vi "S2C_Shared_Proc_GetClusterValues.vi"(4 "LabelText":string, 6 "ClassName":string, 8 "Error In":errorcluster, 9 "CtrlRef":refnum<vi>) -> (0 "Error Out":errorcluster, 2 "Valid?":bool, 3 "Settings":string[](array[string]))   [LabVIEW 2024]
uses:
  <vilib>/Utility/Data Type/NI_Data Type.lvlib
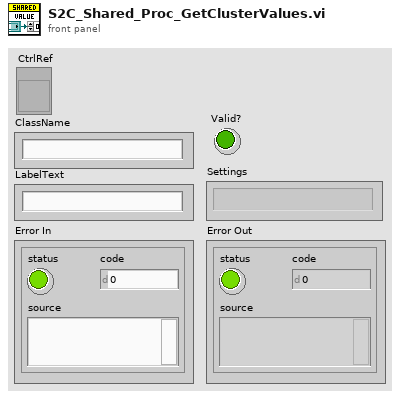
[diagram p1: front panel]
types:
  T1 = typedef "NI_Data Type.lvlib/Data Type.ctl" = enum8{"Invalid Type", "Void", "I8", "I16", "I32", "I64", "U8", "U16", "U32", "U64", "Single Float", "Double Float", "Extended Float", "Single Complex", "Double Complex", "Extended Complex", "Enum U8", "Enum U16", "Enum U32", "Enum U64", "Single Float With Unit", "Double Float With Unit", "Extended Float With Unit", "Single Complex with Unit", "Double Complex with Unit", "Extended Complex with Unit", "Boolean", "String", "Path", "Picture", "Tag", "Array", "Cluster", "Variant", "LV Variant", "Waveform", "Timestamp", "Digital Waveform", "Digital Data", "ExpressData", "Refnum", "External Data", "VI", "Poly VI", "LabVIEW Class Instance", "Fixed Point", "Set Collection", "Map Collection"}
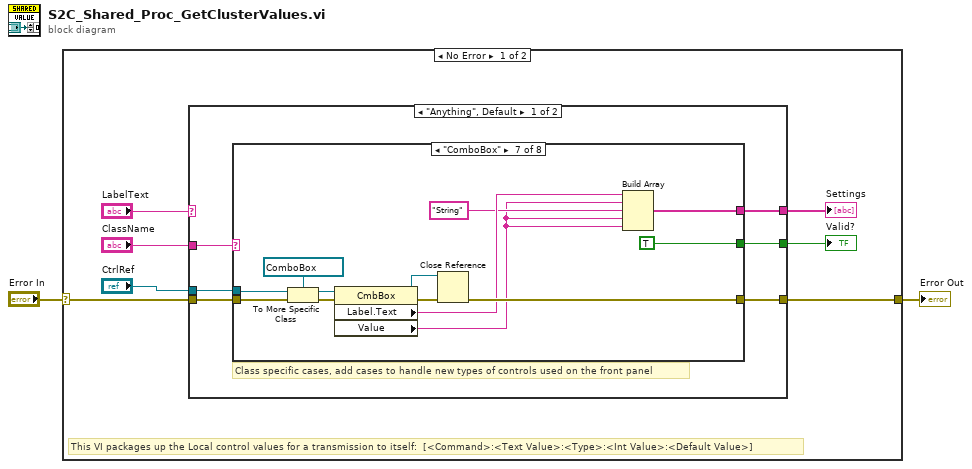
[diagram p0: block diagram]
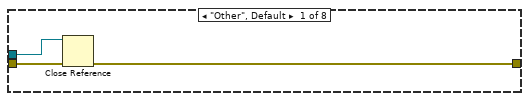
[diagram p2: hidden frame]
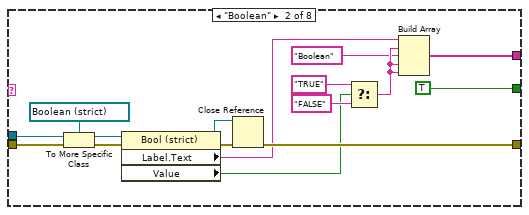
[diagram p3: hidden frame]
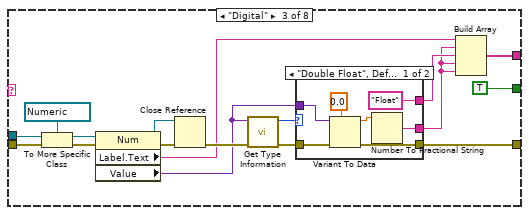
[diagram p4: hidden frame]
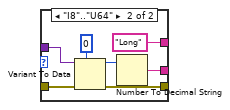
[diagram p5: hidden frame]
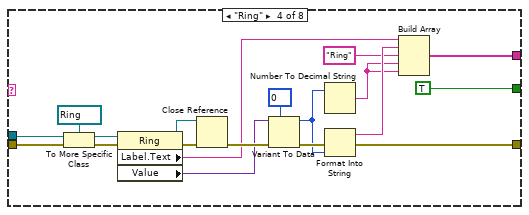
[diagram p6: hidden frame]
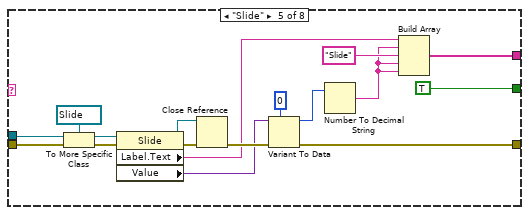
[diagram p7: hidden frame]
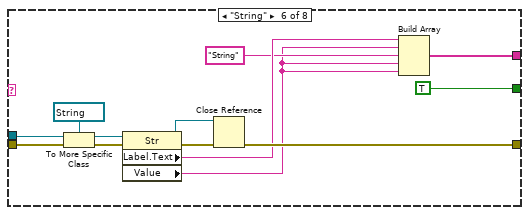
[diagram p8: hidden frame]
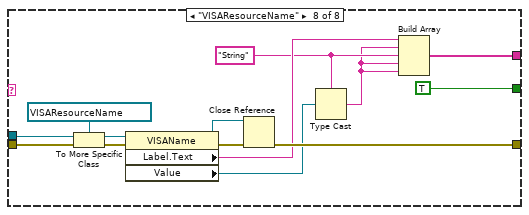
[diagram p9: hidden frame]
diagram:
  n1 = case shown="No Error" "Error In" {
    selector: "Error In" -> [w8 w143]
    tunnel: [w9 w143] -> w1
    frame No Error {
      # "This VI packages up the Local control values for a transmission to itself:  [<Command>:<Text Value>:<Type>:<Int Value>:<Default Value>]"
      n2 = case shown="\"Anything\", Default" "LabelText" {
        tunnel: [w15 w142] -> w9
        tunnel: w8 -> [w14 w142]
        tunnel: "CtrlRef" -> [w13 _]
        tunnel: [w12 _] -> w6
        tunnel: [w11 _] -> w5
        tunnel: "ClassName" -> [w10 _]
        frame "Anything", Default {
          # "Class specific cases, add cases to handle new types of controls used on the front panel"
          n3 = case shown="\"ComboBox\"" w10 {
            tunnel: w14 -> [w18 w34 w51 w84 w101 w114 w127 w141]
            tunnel: w13 -> [w16 w33 w50 w83 w100 w113 w126 w140]
            tunnel: [_ w26 w46 w78 w95 w108 w121 w135] -> w12
            tunnel: [w17 w23 w38 w71 w85 w105 w118 w132] -> w15
            tunnel: [_ TRUE TRUE TRUE TRUE TRUE TRUE TRUE] -> w11
            frame "Other", Default {
              n4 = Close Reference(reference=w16, error in (no error)=w18) -> (error out=w17:errorcluster)
            }
            frame "Boolean" {
              n5 = To More Specific Class(target class=refnum<vi> refnum ("reference"), reference=w33, error in=w34) -> (specific class reference=w31:refnum<vi>, error out=w32:errorcluster)
              n6 = property class="Bool (strict)"(reference=w31, error in=w32) -> (reference out=w29:refnum<vi>, error out=w30:errorcluster, "Label.Text"=w21:string, "Value"=w22:bool)
              n7 = Close Reference(reference=w29, error in (no error)=w30) -> (error out=w23:errorcluster)
              n8 = Select(t="TRUE", s=w22, f="FALSE") -> (s? t:f=w20:string)
              n9 = Build Array(w21, w20, "Boolean" ("element"), w20, w20) -> (w26:string[])
            }
            frame "Digital" {
              n10 = To More Specific Class(target class=refnum<vi> refnum ("reference"), reference=w50, error in=w51) -> (specific class reference=w43:refnum<vi>, error out=w49:errorcluster)
              n11 = property class="Num"(reference=w43, error in=w49) -> (reference out=w47:refnum<vi>, error out=w48:errorcluster, "Label.Text"=w37:string, "Value"=w39:variant)
              n12 = Close Reference(reference=w47, error in (no error)=w48) -> (error out=w42:errorcluster)
              n13 = call <vilib>:"Get Type Information.vi"("error in (no error)"=w42, "variant"=w39) -> ("error out"=w41:errorcluster, "type"=w40:T1)  [unwired: 5 in, 3 out]
              n14 = case shown="\"Double Float\", Default" w40 {
                tunnel: w41 -> [w58 w65]
                tunnel: w39 -> [w56 w63]
                tunnel: [w55 w62] -> w38
                tunnel: [w53 w60] -> w35
                tunnel: ["Float" "Long"] -> w36
                frame "Double Float", Default {
                  n15 = Variant To Data(error in=w58, type=0.0, Variant=w56) -> (data=w54:dbl, error out=w55:errorcluster)
                  n16 = Number To Fractional String(number=w54) -> (F-format string=w53:string)  [unwired: 3 in]
                }
                frame "I8".."U64" {
                  n17 = Variant To Data(error in=w65, type=0, Variant=w63) -> (data=w61:i32, error out=w62:errorcluster)
                  n18 = Number To Decimal String(number=w61) -> (decimal integer string=w60:string)  [unwired: 1 in]
                }
              }
              n19 = Build Array(w37, w35, w36, w35, w35) -> (w46:string[])
            }
            frame "Ring" {
              w66 = u16 0 items=[""]
              n20 = To More Specific Class(target class=refnum<vi> refnum ("reference"), reference=w83, error in=w84) -> (specific class reference=w81:refnum<vi>, error out=w82:errorcluster)
              n21 = property class="Ring"(reference=w81, error in=w82) -> (reference out=w79:refnum<vi>, error out=w80:errorcluster, "Label.Text"=w73:string, "Value"=w74:variant)
              n22 = Close Reference(reference=w79, error in (no error)=w80) -> (error out=w75:errorcluster)
              n23 = Variant To Data(error in=w75, type=w66, Variant=w74) -> (data=w70:u16, error out=w72:errorcluster)
              n24 = Number To Decimal String(number=w70) -> (decimal integer string=w67:string)  [unwired: 1 in]
              n25 = Format Into String(error in=w72, w70) -> (resulting string=w69:string, error out=w71:errorcluster)  [unwired: 2 in]
              n26 = Build Array(w73, w69, "Ring" ("element"), w67, w67) -> (w78:string[])
            }
            frame "Slide" {
              n27 = To More Specific Class(target class=refnum<vi> refnum ("reference"), reference=w100, error in=w101) -> (specific class reference=w98:refnum<vi>, error out=w99:errorcluster)
              n28 = property class="Slide"(reference=w98, error in=w99) -> (reference out=w96:refnum<vi>, error out=w97:errorcluster, "Label.Text"=w90:string, "Value"=w91:variant)
              n29 = Close Reference(reference=w96, error in (no error)=w97) -> (error out=w92:errorcluster)
              n30 = Variant To Data(error in=w92, type=0 ("Scan1"), Variant=w91) -> (data=w89:i32, error out=w85:errorcluster)
              n31 = Number To Decimal String(number=w89) -> (decimal integer string=w86:string)  [unwired: 1 in]
              n32 = Build Array(w90, w86, "Slide" ("element"), w86, w86) -> (w95:string[])
            }
            frame "String" {
              n33 = To More Specific Class(target class=refnum<vi> refnum ("reference"), reference=w113, error in=w114) -> (specific class reference=w111:refnum<vi>, error out=w112:errorcluster)
              n34 = property class="Str"(reference=w111, error in=w112) -> (reference out=w109:refnum<vi>, error out=w110:errorcluster, "Label.Text"=w104:string, "Value"=w102:string)
              n35 = Close Reference(reference=w109, error in (no error)=w110) -> (error out=w105:errorcluster)
              n36 = Build Array(w104, w102, "String" ("element"), w102, w102) -> (w108:string[])
            }
            frame "ComboBox" {
              n37 = To More Specific Class(target class=refnum<vi> refnum ("reference"), reference=w126, error in=w127) -> (specific class reference=w124:refnum<vi>, error out=w125:errorcluster)
              n38 = property class="CmbBox"(reference=w124, error in=w125) -> (reference out=w122:refnum<vi>, error out=w123:errorcluster, "Label.Text"=w117:string, "Value"=w115:string)
              n39 = Close Reference(reference=w122, error in (no error)=w123) -> (error out=w118:errorcluster)
              n40 = Build Array(w117, w115, "String" ("element"), w115, w115) -> (w121:string[])
            }
            frame "VISAResourceName" {
              w130 = "String" ("element")
              n41 = To More Specific Class(target class=refnum<vi> refnum ("reference"), reference=w140, error in=w141) -> (specific class reference=w138:refnum<vi>, error out=w139:errorcluster)
              n42 = property class="VISAName"(reference=w138, error in=w139) -> (reference out=w136:refnum<vi>, error out=w137:errorcluster, "Label.Text"=w131:string, "Value"=w129:refnum<visa-resource-name>)
              n43 = Close Reference(reference=w136, error in (no error)=w137) -> (error out=w132:errorcluster)
              n44 = Type Cast(type=w130, x=w129) -> (*(type *) &x=w128:string)
              n45 = Build Array(w131, w128, w130, w128, w128) -> (w135:string[])
            }
          }
        }
        frame "P1C1Exe".."P8C8Exe" {
          # "This case handles the \"Execute\" buttons"
        }
      }
      "Settings" <- w6
      "Valid?" <- w5
    }
    frame Error {
    }
  }
  "Error Out" <- w1
